vi "Shooting Managment.vi"(0 "Start Shooting Procedure":bool) -> (1 "Disable Stack Ordering":bool, 2 "Is Shooting?":bool)   [LabVIEW 2012]
uses:
  BotStatus.vi
  Motors Values.vi
panel:
  # "ADD Override!!!!!!!!!!!!!!!!!!!!!!!!"
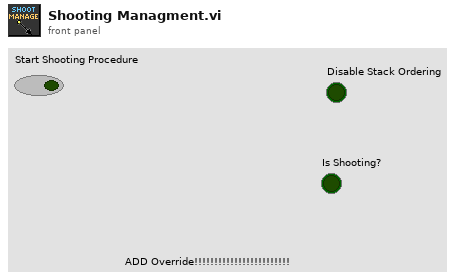
[diagram p1: front panel]
types:
  T1 = cluster{"Middle":bool, "Cannon":bool, "InFlipper":bool, "FlipperAtPlace":bool, "Bottom":bool, "FrisbeeDirection":bool}
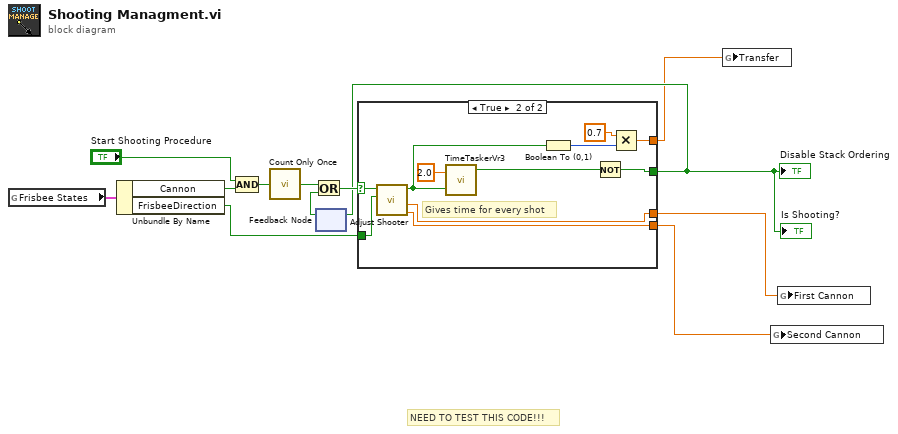
[diagram p0: block diagram]
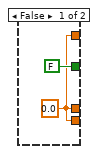
[diagram p2: hidden frame]
diagram:
  # "NEED TO TEST THIS CODE!!!"
  n1 = global read "BotStatus.vi" "Frisbee States"() -> (w8:T1)
  n2 = Unbundle By Name(w8) -> ("Cannon"=w6:bool, "FrisbeeDirection"=w7:bool)
  n3 = Compound Arithmetic op=AND("Start Shooting Procedure", w6) -> (w5:bool)
  n4 = call "Count Only Once.vi"("InValue"=w5) -> ("Result"=w11:bool)
  n5 = feedback #1() -> (w10:bool)  [unwired: 1 in]
  n6 = Or(x=w11, y=w10) -> (x .or. y?=w12:bool)
  n7 = case shown="True" w12 {
    selector: w12 -> [_ w18]
    tunnel: [FALSE ("READY!") w19] -> w4
    tunnel: [w13 w23] -> w1
    tunnel: [w13 w17] -> w3
    tunnel: [w13 w16] -> w2
    tunnel: w7 -> [_ w15]
    frame False {
      w13 = 0.0
    }
    frame True {
      # "Gives time for every shot"
      n8 = call "Adjust Shooter.vi"("Upside Down?"=w15, "Start to Adjust"=w18) -> ("Second Cannon"=w16:dbl, "First Cannon"=w17:dbl, "READY!"=w21:bool)  [unwired: 2 in, 1 out]
      n9 = call "TimeTaskerVr3.vi"("Delay(sec)"=2.0, "Start Counting?"=w21) -> ("TimePast?"=w20:bool)  [unwired: 2 out]
      n10 = Boolean To (0,1)(Boolean=w21) -> (0, 1=w25:i16)
      n11 = Not(x=w20) -> (.not. x?=w19:bool)
      n12 = Multiply(x=0.7, y=w25) -> (x*y=w23:dbl)
    }
  }
  "Disable Stack Ordering" <- w4
  "Is Shooting?" <- w4
  n13 = feedback-in #1(w4) -> ()
  n14 = global write "Motors Values.vi" "Transfer"(w1) -> ()
  n15 = global write "Motors Values.vi" "Second Cannon"(w2) -> ()
  n16 = global write "Motors Values.vi" "First Cannon"(w3) -> ()
